vi "Instrument fgv uno.vi"(7 "Enum":T1(ring), 8 "error in (no error) 2":errorcluster, 9 "milliseconds to wait":u32=60, 10 "WriteCC1":string[](array[string])=[""], 11 "INPUT":T2) -> (0 "error":errorcluster, 2 "WriteCC1 2":string[](array[string]), 3 "output":T2)   [LabVIEW 2025]
uses:
  cf2ff1be-2106-4981-a75b-2e942dcf7eff.vi
  <vilib>/Instr/_visa.llb/VISA Configure Serial Port (Instr).vi
panel:
  out "error out 2":errorcluster
  out "error out":errorcluster
  out "error out":errorcluster
  out "Serial Settings:Number of Bytes at Serial Port":u32
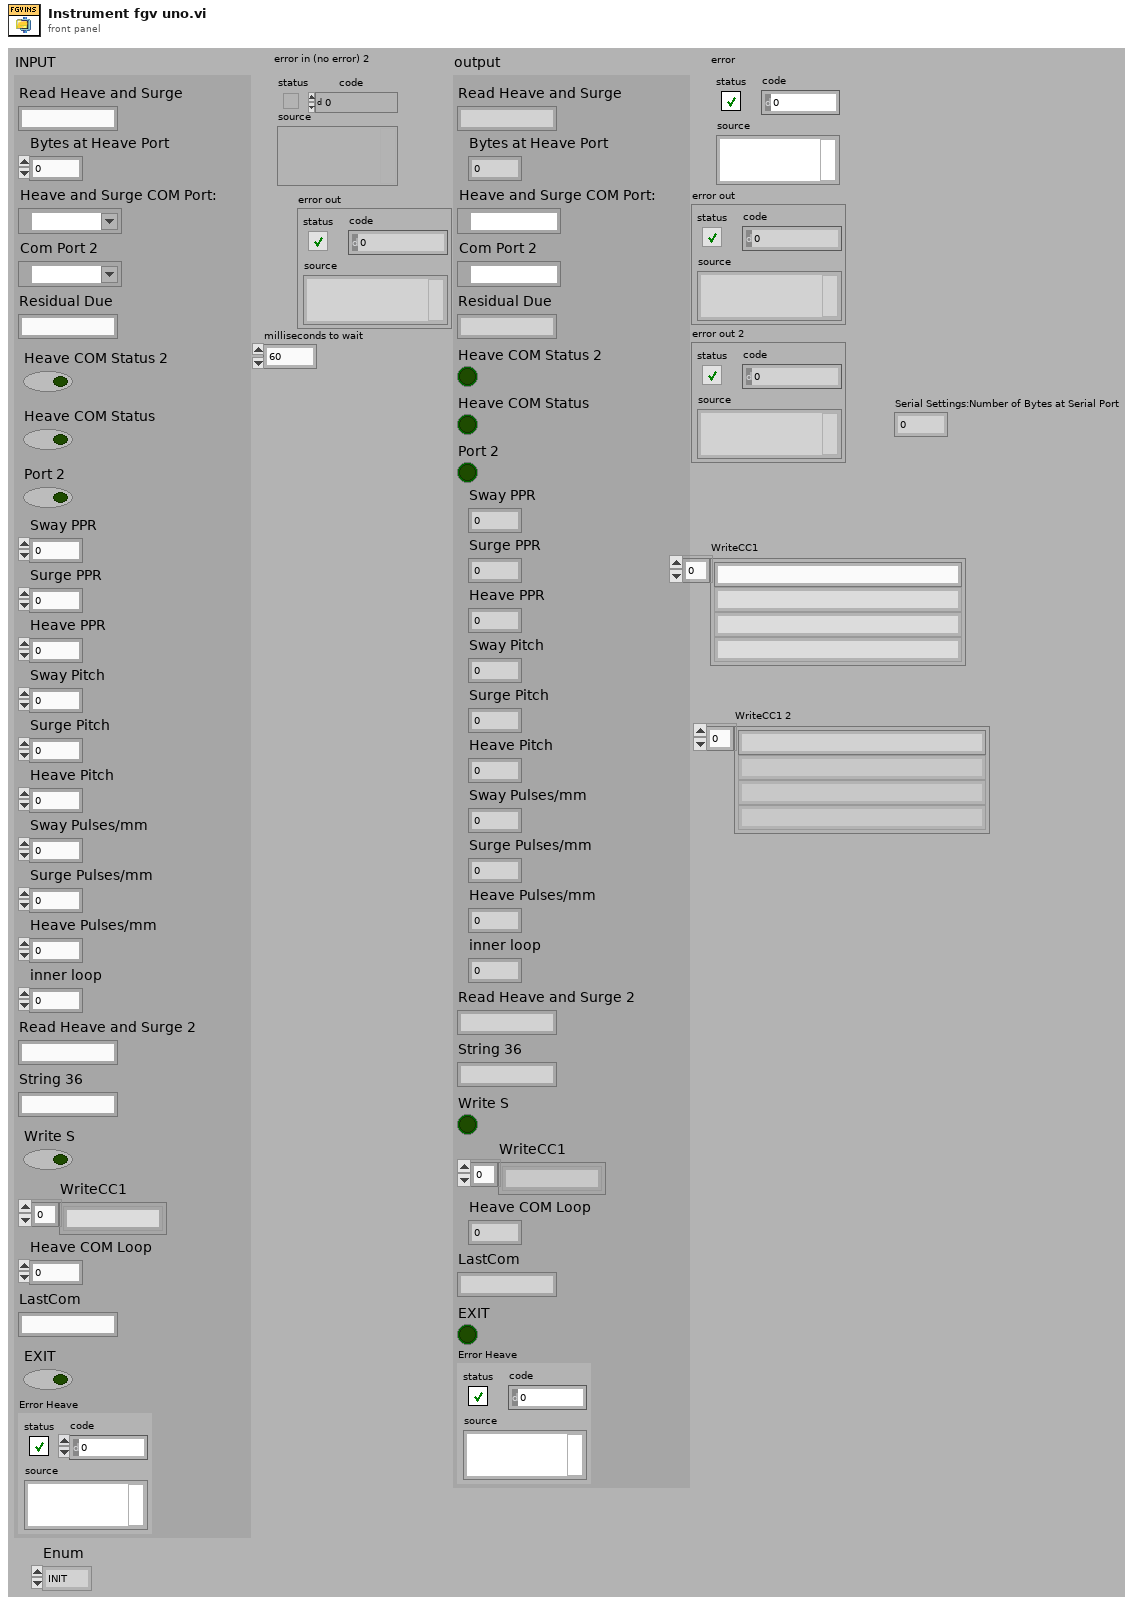
[diagram p1: front panel]
types:
  T1 = enum16{"INIT", "READ", "MANUAL WRITE", "WRITE", "CLOSE", "ERROR INIT"}
  T2 = cluster{"Read Heave and Surge":string, "Bytes at Heave Port":dbl, "Heave and Surge COM Port:":refnum<visa-resource-name>, "Com Port 2":refnum<visa-resource-name>, "Residual Due":string, "Heave COM Status 2":bool, "Heave COM Status":bool, "Port 2":bool, "Sway PPR":dbl, "Surge PPR":dbl, "Heave PPR":dbl, "Sway Pitch":dbl, "Surge Pitch":dbl, "Heave Pitch":dbl, "Sway Pulses/mm":dbl, "Surge Pulses/mm":dbl, "Heave Pulses/mm":dbl, "inner loop":dbl, "Read Heave and Surge 2":string, "String 36":string, "Write S":bool, "WriteCC1":string[], "Heave COM Loop":i32, "LastCom":string, "EXIT":bool, "Error Heave":errorcluster}
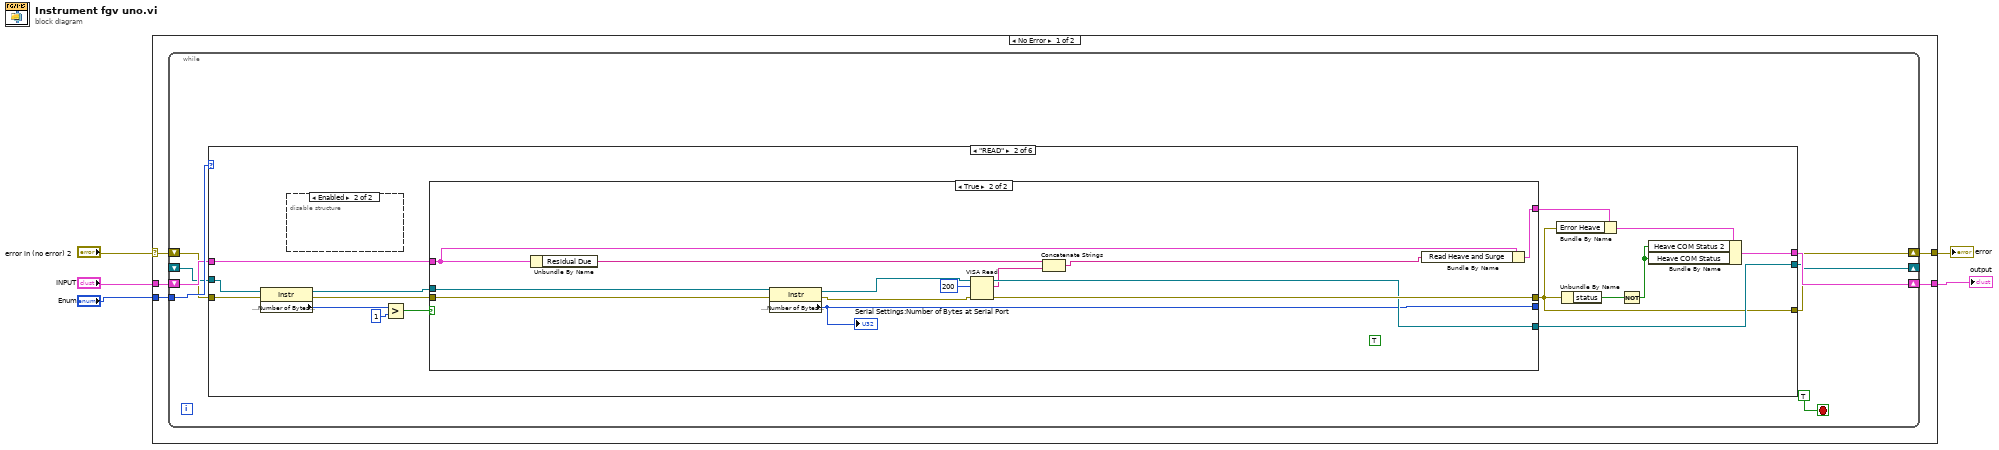
[diagram p0: block diagram]
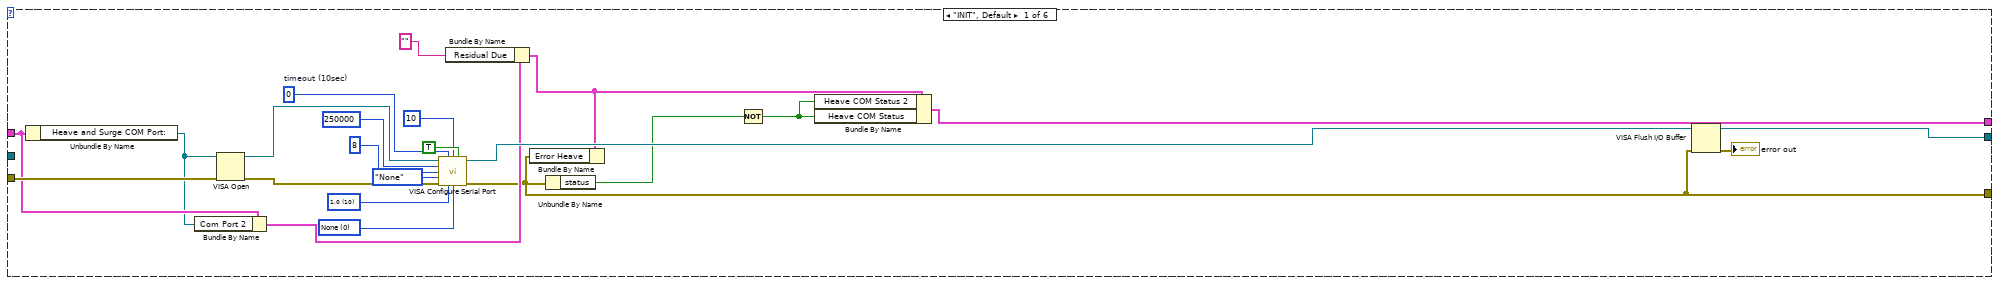
[diagram p2: hidden frame]
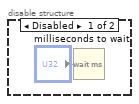
[diagram p3: hidden frame]
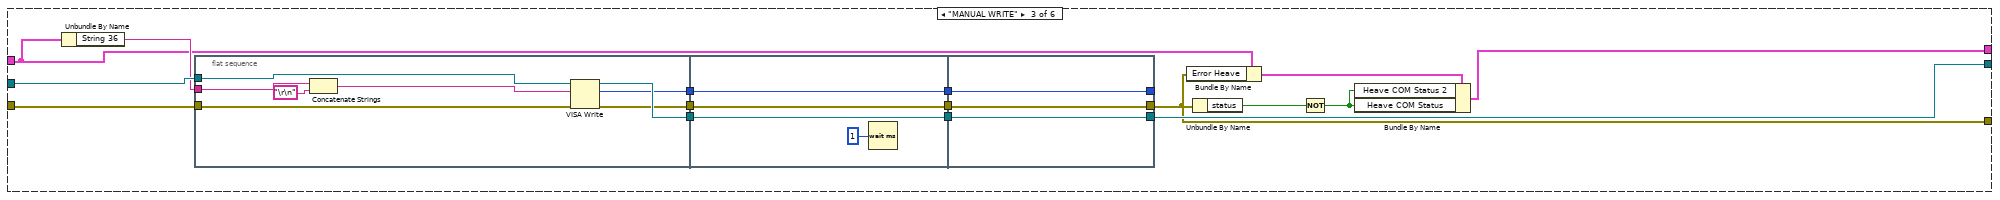
[diagram p5: hidden frame]
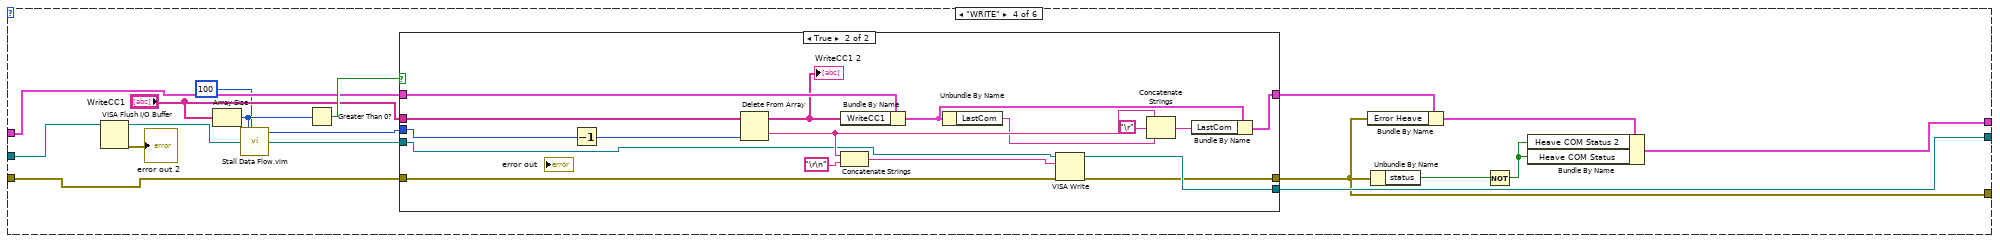
[diagram p6: hidden frame]
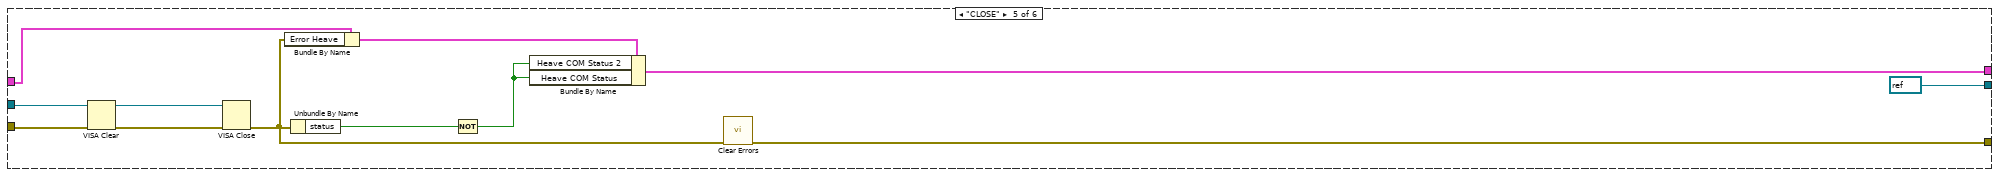
[diagram p8: hidden frame]
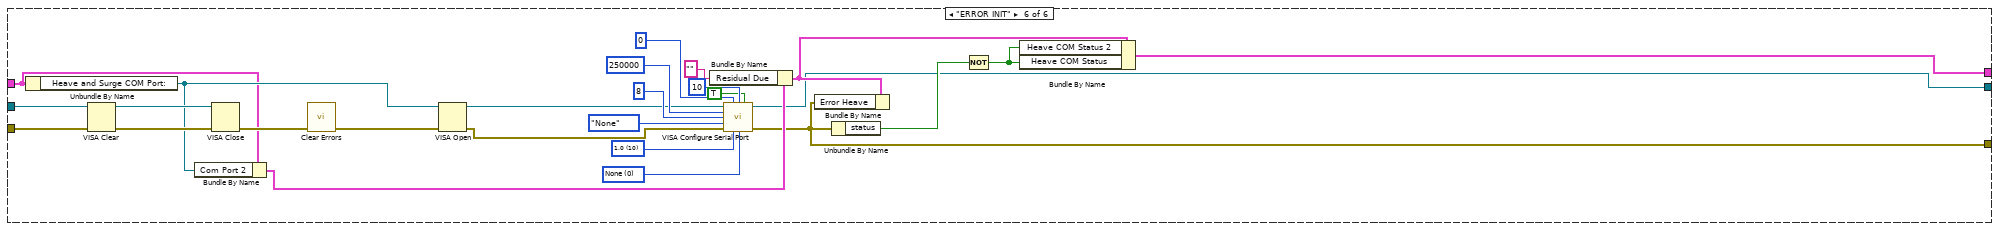
[diagram p9: hidden frame]
diagram:
  n1 = case shown="No Error" "error in (no error) 2" {
    selector: "error in (no error) 2" -> [w9 w180]
    tunnel: [w10 w180] -> w2
    tunnel: "Enum" -> [w8 _]
    tunnel: "INPUT" -> [w7 w181]
    tunnel: [w6 w181] -> w5
    frame No Error {
      n2 = while {
        tunnel: w8 -> [w17]
        shift-right: [w13] -> w10
        shift-left: w9 -> [w14]
        shift-right: [w16] -> w6
        shift-left: w7 -> [w15]
        shift-right: [w12] -> _
        shift-left: _ -> [w11]
        stop <- TRUE ("stop 3") stop-if-true
        n3 = case shown="\"READ\"" w17 {
          tunnel: [w31 w45 w75 w114 w143 w157] -> w16
          tunnel: w15 -> [w27 w49 w77 w117 w144 w161]
          tunnel: w14 -> [w28 w56 w81 w119 w151 w176]
          tunnel: [w23 w42 w76 w113 w149 w159] -> w13
          tunnel: [w24 w44 w82 w118 refnum<visa-resource-name> refnum ("duplicate VISA resource name") w158] -> w12
          tunnel: w11 -> [_ w55 w83 w109 w150 w175]
          frame "INIT", Default {
            w40 = u16 0 items=["None", "XON/XOFF", "RTS/CTS", "XON/XOFF & RTS/CTS", "DTR/DSR", "XON/XOFF & DTR/DSR"] ("flow control (0:none)  2")
            w38 = u16 10 items=["1.0"=10, "1.5"=15, "2.0"=20] ("stop bits 2")
            w36 = u32 0  # timeout (10sec)
            n4 = Unbundle By Name(w27) -> ("Heave and Surge COM Port:"=w25:refnum<visa-resource-name>)
            n5 = Bundle By Name(cluster=w27, "Com Port 2"=w25) -> (w26:T2)
            n6 = VISA Open(error in (no error)=w28, VISA resource name=w25) -> (VISA resource name=w34:refnum<visa-resource-name>, error out=w35:errorcluster)  [unwired: 3 in]
            n7 = call-poly "VISA Configure Serial Port"("VISA resource name"=w34, "timeout (10sec)"=w36, "termination char\n(0xA = '\\n' = LF)"=u8 10 ("termination char\n(0xA = '\\n' = LF)"), "Enable Termination\nChar (T)"=TRUE ("Enable Termination\nChar (T)"), "baud rate (9600)"=u32 250000 ("baud rate  2"), "data bits (8)"=u16 8 ("data bits  2"), "parity (0:none)"=enum16{"None", "Odd", "Even", "Mark", "Space"}."None", "error in (no error)"=w35, "stop bits (10: 1 bit)"=w38, "flow control (0:none)"=w40) -> ("VISA resource name out"=w33:refnum<visa-resource-name>, "error out"=w23:errorcluster)  [unwired: 4 in]
            n8 = Bundle By Name(cluster=w26, "Residual Due"="") -> (w32:T2)
            n9 = Bundle By Name(cluster=w32, "Error Heave"=w23) -> ()  [unwired: 1 out]
            n10 = Unbundle By Name(w23) -> ("status"=w30:bool)
            n11 = Not(x=w30) -> (.not. x?=w29:bool)
            n12 = Bundle By Name(cluster=w32, "Heave COM Status 2"=w29, "Heave COM Status"=w29) -> (w31:T2)
            n13 = VISA Flush I/O Buffer(VISA resource name=w33, error in (no error)=w23) -> (VISA resource name out=w24:refnum<visa-resource-name>, error out=→"error out":errorcluster)  [unwired: 1 in]
          }
          frame "READ" {
            n14 = property class="Instr"(reference=w55, error in=w56) -> (reference out=w51:refnum<visa-resource-name>, error out=w50:errorcluster, "Serial Settings:Number of Bytes at Serial Port"=w54:u32)
            n15 = disable-structure shown="Enabled" {
              frame Disabled {
                n16 = Wait (ms)(milliseconds to wait="milliseconds to wait") -> ()  [unwired: 1 out]
              }
              frame Enabled {
              }
            }
            n17 = Greater?(x=w54, y=u32 1) -> (0:w52:bool)
            n18 = case shown="True" w52 {
              tunnel: w51 -> [w60 w70]
              tunnel: w50 -> [w59 w71]
              tunnel: [w59 w73] -> w42
              tunnel: [w60 w72] -> w44
              tunnel: w49 -> [w58 w69]
              tunnel: [w58 w67] -> w48
              tunnel: [_ w62] -> _
              frame False {
              }
              frame True {
                (unwired) TRUE
                n19 = Unbundle By Name(w69) -> ("Residual Due"=w68:string)
                n20 = property class="Instr"(reference=w70, error in=w71) -> (reference out=w65:refnum<visa-resource-name>, error out=w64:errorcluster, "Serial Settings:Number of Bytes at Serial Port"=w62:u32)
                "Serial Settings:Number of Bytes at Serial Port" <- w62
                n21 = VISA Read(VISA resource name=w65, byte count=u32 200, error in (no error)=w64) -> (VISA resource name out=w72:refnum<visa-resource-name>, read buffer=w63:string, error out=w73:errorcluster)  [unwired: 1 out]
                n22 = Concatenate Strings(w68, w63) -> (w66:string)
                n23 = Bundle By Name(cluster=w69, "Read Heave and Surge"=w66) -> (w67:T2)
              }
            }
            n24 = Bundle By Name(cluster=w48, "Error Heave"=w42) -> (w47:T2)
            n25 = Unbundle By Name(w42) -> ("status"=w46:bool)
            n26 = Not(x=w46) -> (.not. x?=w43:bool)
            n27 = Bundle By Name(cluster=w47, "Heave COM Status 2"=w43, "Heave COM Status"=w43) -> (w45:T2)
          }
          frame "MANUAL WRITE" {
            n28 = Unbundle By Name(w77) -> ("String 36"=w80:string)
            n29 = flat-sequence {
              tunnel: w83 -> [w94]
              tunnel: w81 -> [w93]
              tunnel: w80 -> [w92]
              tunnel: [w97] -> w89
              tunnel: [w96] -> w88
              tunnel: [w95] -> w87
              tunnel: w89 -> [w101]
              tunnel: w88 -> [w100]
              tunnel: w87 -> [w99]
              tunnel: [w101] -> w86
              tunnel: [w100] -> w85
              tunnel: [w99] -> w84
              tunnel: [w102] -> _
              tunnel: [w103] -> w76
              tunnel: [w104] -> w82
              tunnel: w86 -> [w104]
              tunnel: w85 -> [w103]
              tunnel: w84 -> [w102]
              frame #0 {
                n30 = Concatenate Strings(w92, "\r\n") -> (w91:string)
                n31 = VISA Write(VISA resource name=w94, write buffer=w91, error in (no error)=w93) -> (VISA resource name out=w97:refnum<visa-resource-name>, return count=w95:u32, error out=w96:errorcluster)
              }
              frame #1 {
                n32 = Wait (ms)(milliseconds to wait=u32 1) -> ()  [unwired: 1 out]
              }
              frame #2 {
              }
            }
            n33 = Bundle By Name(cluster=w77, "Error Heave"=w76) -> (w79:T2)
            n34 = Unbundle By Name(w76) -> ("status"=w78:bool)
            n35 = Not(x=w78) -> (.not. x?=w74:bool)
            n36 = Bundle By Name(cluster=w79, "Heave COM Status 2"=w74, "Heave COM Status"=w74) -> (w75:T2)
          }
          frame "WRITE" {
            n37 = VISA Flush I/O Buffer(VISA resource name=w109) -> (VISA resource name out=w108:refnum<visa-resource-name>, error out=→"error out 2":errorcluster)  [unwired: 2 in]
            n38 = Array Size(array="WriteCC1") -> (size(s)=w121:i32)
            n39 = call "Stall Data Flow.vim"("value in"=w108, "milliseconds to wait"=u32 100) -> ("value out"=w106:refnum<visa-resource-name>)  [unwired: 1 out]
            n40 = Greater Than 0?(x=w121) -> (x > 0?=w120:bool)
            n41 = case shown="True" w120 {
              tunnel: [w124 w135] -> w113
              tunnel: w119 -> [w124 w140]
              tunnel: [w122 w139] -> w118
              tunnel: "WriteCC1" -> [_ w136]
              tunnel: w121 -> [_ w138]
              tunnel: w117 -> [w123 w132]
              tunnel: [w123 w129] -> w116
              tunnel: w106 -> [w122 w125]
              frame False {
              }
              frame True {
                n42 = Decrement(x=w138) -> (x-1=w137:i32)
                n43 = Delete From Array(array=w136, index=w137) -> (deleted portion=w134:string, array with subset deleted=w128:string[])  [unwired: 1 in]
                "WriteCC1 2" <- w128
                n44 = Bundle By Name(cluster=w132, "WriteCC1"=w128) -> (w131:T2)
                n45 = Concatenate Strings(w134, "\r\n") -> (w127:string)
                n46 = Unbundle By Name(w131) -> ("LastCom"=w130:string)
                n47 = VISA Write(VISA resource name=w125, write buffer=w127, error in (no error)=w140) -> (VISA resource name out=w139:refnum<visa-resource-name>, error out=w135:errorcluster)  [unwired: 1 out]
                n48 = Concatenate Strings(w134, "\r", w130) -> (w133:string)
                n49 = Bundle By Name(cluster=w131, "LastCom"=w133) -> (w129:T2)
              }
            }
            n50 = Bundle By Name(cluster=w116, "Error Heave"=w113) -> (w115:T2)
            n51 = Unbundle By Name(w113) -> ("status"=w112:bool)
            n52 = Not(x=w112) -> (.not. x?=w111:bool)
            n53 = Bundle By Name(cluster=w115, "Heave COM Status 2"=w111, "Heave COM Status"=w111) -> (w114:T2)
          }
          frame "CLOSE" {
            n54 = VISA Clear(VISA resource name=w150, error in (no error)=w151) -> (VISA resource name out=w153:refnum<visa-resource-name>, error out=w152:errorcluster)
            n55 = VISA Close(VISA resource name=w153, error in (no error)=w152) -> (error out=w145:errorcluster)
            n56 = Bundle By Name(cluster=w144, "Error Heave"=w145) -> (w148:T2)
            n57 = Unbundle By Name(w145) -> ("status"=w147:bool)
            n58 = Not(x=w147) -> (.not. x?=w146:bool)
            n59 = Bundle By Name(cluster=w148, "Heave COM Status 2"=w146, "Heave COM Status"=w146) -> (w143:T2)
            n60 = call <vilib>:"Clear Errors.vi"("error in (no error)"=w145) -> ("error out"=w149:errorcluster)  [unwired: 5 in, 1 out]
          }
          frame "ERROR INIT" {
            w173 = u16 0 items=["None", "XON/XOFF", "RTS/CTS", "XON/XOFF & RTS/CTS", "DTR/DSR", "XON/XOFF & DTR/DSR"] ("flow control (0:none)  2")
            w171 = u16 10 items=["1.0"=10, "1.5"=15, "2.0"=20] ("stop bits 2")
            n61 = Unbundle By Name(w161) -> ("Heave and Surge COM Port:"=w162:refnum<visa-resource-name>)
            n62 = VISA Clear(VISA resource name=w175, error in (no error)=w176) -> (VISA resource name out=w179:refnum<visa-resource-name>, error out=w178:errorcluster)
            n63 = Bundle By Name(cluster=w161, "Com Port 2"=w162) -> (w163:T2)
            n64 = VISA Close(VISA resource name=w179, error in (no error)=w178) -> (error out=w177:errorcluster)
            n65 = call <vilib>:"Clear Errors.vi"("error in (no error)"=w177) -> ("error out"=w160:errorcluster)  [unwired: 5 in, 1 out]
            n66 = VISA Open(error in (no error)=w160, VISA resource name=w162) -> (VISA resource name=w167:refnum<visa-resource-name>, error out=w168:errorcluster)  [unwired: 3 in]
            n67 = Bundle By Name(cluster=w163, "Residual Due"="") -> (w166:T2)
            n68 = call-poly "VISA Configure Serial Port"("VISA resource name"=w167, "timeout (10sec)"=u32 0, "termination char\n(0xA = '\\n' = LF)"=u8 10 ("termination char\n(0xA = '\\n' = LF)"), "Enable Termination\nChar (T)"=TRUE ("Enable Termination\nChar (T)"), "baud rate (9600)"=u32 250000 ("baud rate  2"), "data bits (8)"=u16 8 ("data bits  2"), "parity (0:none)"=enum16{"None", "Odd", "Even", "Mark", "Space"}."None", "error in (no error)"=w168, "stop bits (10: 1 bit)"=w171, "flow control (0:none)"=w173) -> ("VISA resource name out"=w158:refnum<visa-resource-name>, "error out"=w159:errorcluster)  [unwired: 4 in]
            n69 = Bundle By Name(cluster=w166, "Error Heave"=w159) -> ()  [unwired: 1 out]
            n70 = Unbundle By Name(w159) -> ("status"=w165:bool)
            n71 = Not(x=w165) -> (.not. x?=w164:bool)
            n72 = Bundle By Name(cluster=w166, "Heave COM Status 2"=w164, "Heave COM Status"=w164) -> (w157:T2)
          }
        }
      }
    }
    frame Error {
    }
  }
  "output" <- w5
  "error" <- w2
